vi "folder&single VI desc&help.vi"() -> ()   [LabVIEW 2020]
panel:
  in  "All / Selected by Name":bool
  in  "Same Desc":bool
  in  "Copy Descs to Tags":bool
  in  "PREV":bool
  in  "NEXT":bool
  out "filenames":string[](array[string])
  in  "Read entire Folder":bool
  in  "path":path
  in  "stop":bool
  in  "SAVE":bool
  in  "Copy Desc&Tags":bool
  in  "Same File":bool
  out "found index":i32[](array[numeric])
  in  "Select Name":string[](array[string])
  in  "Copy VI Descr W":bool
  in  "Tip W":string[](array[string])
  in  "Desc W":string[](array[string])
  out "Is Ind?":bool[](array[boolean])
  out "Desc":string[](array[string])
  out "Tip":string[](array[string])
  out "Name":string[](array[string])
  out "index":i32[](array[numeric])
  out "ClassID":u32[](array[numeric])
  out "ClassName":string[](array[string])
  in  "Generate Help Tag W":bool
  in  "Copy Help Tag":bool
  in  "Copy CHM path":bool
  in  "W vi path":path
  in  "Help:Document Path W":path
  in  "Help:Document Tag W":string
  in  "VI Description W":string
  out "VI Name W":string
  in  "Write":bool
  in  "Read":bool
  out "VI Name":string
  out "VI Description":string
  out "Help:Document Tag":string
  out "Help:Document Path":path
  in  "R vi path":path
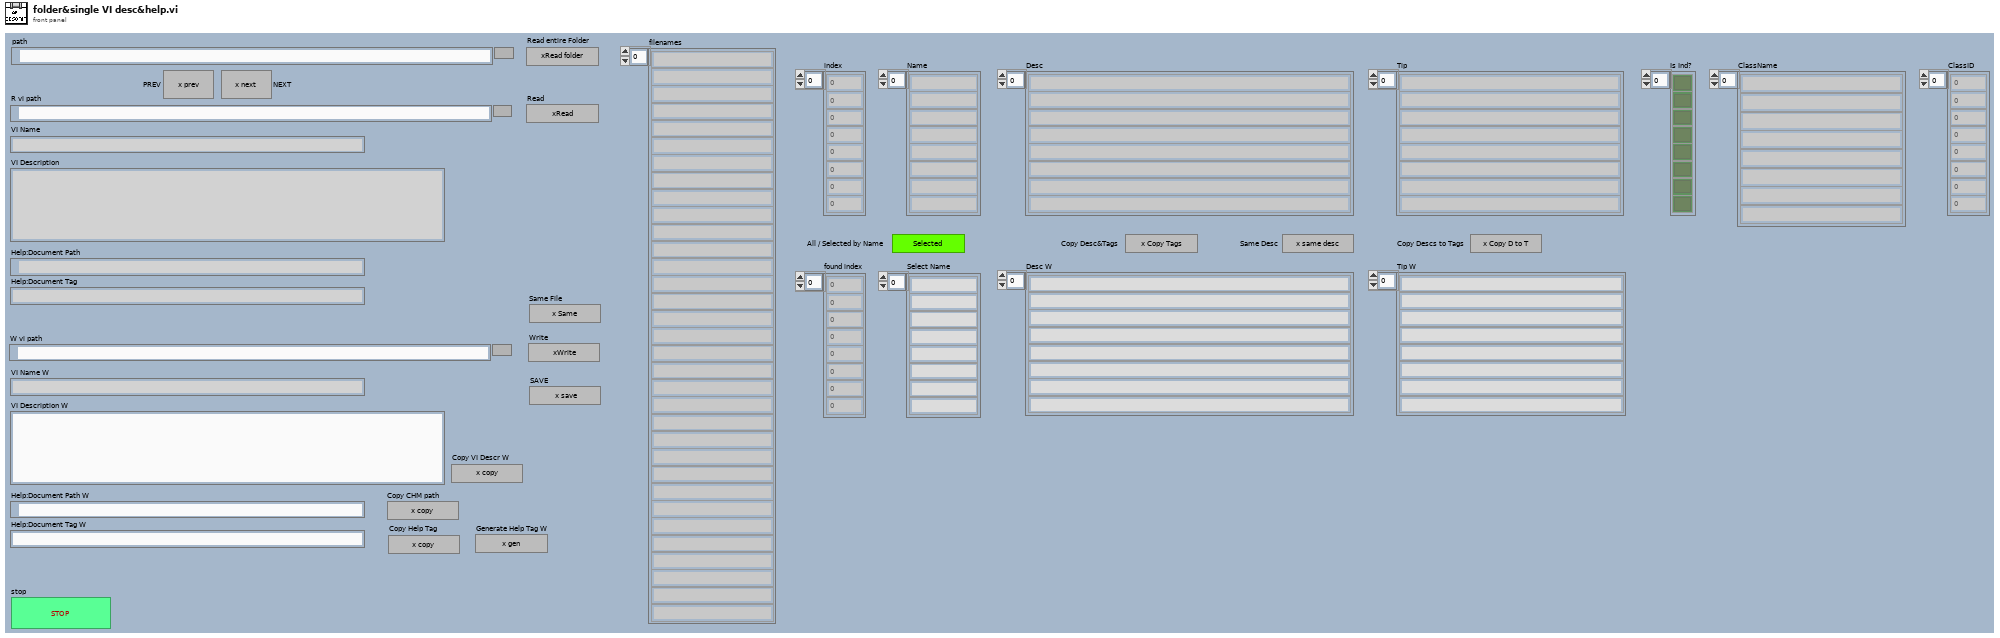
[diagram p1: front panel]
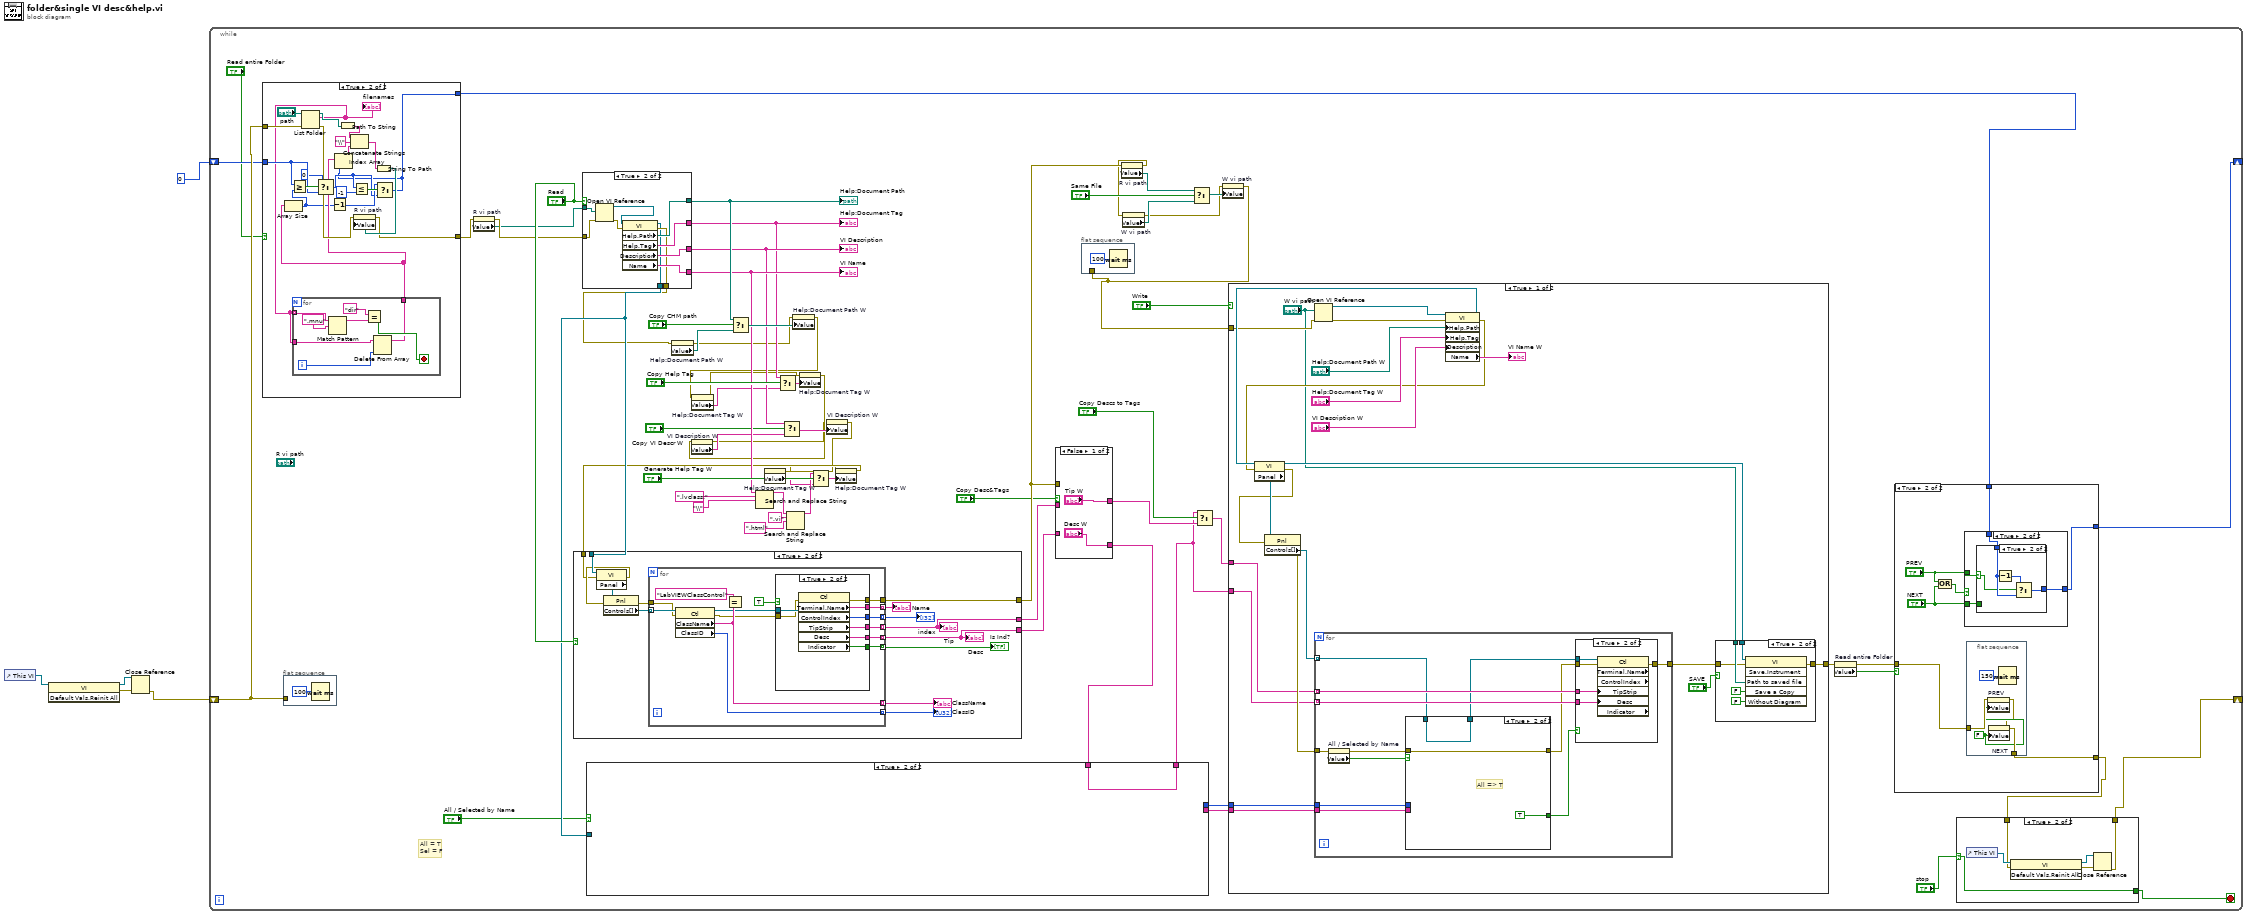
[diagram p0: block diagram]
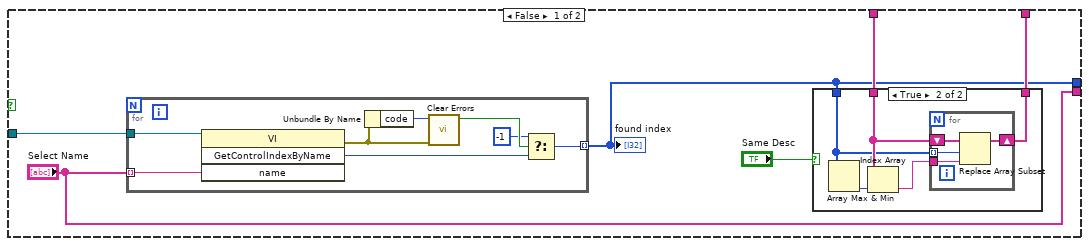
[diagram p2: hidden frame]
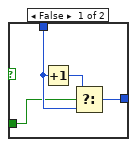
[diagram p8: hidden frame]
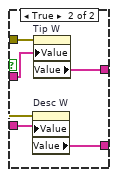
[diagram p9: hidden frame]
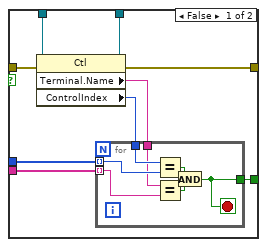
[diagram p11: hidden frame]
diagram:
  n1 = control-ref of="This VI"() -> (w4:refnum<vi>)
  n2 = invoke class="VI" method="Default Vals.Reinit All"(reference=w4) -> (reference out=w2:refnum<vi>, error out=w3:errorcluster)  [unwired: 2 in, 1 out]
  n3 = Close Reference(reference=w2, error in (no error)=w3) -> (error out=w1:errorcluster)
  n4 = while {
    shift-right: [w28] -> _
    shift-left: w1 -> [w72]
    shift-right: [w73] -> _
    shift-left: 0 -> [w71]
    stop <- w30 stop-if-true
    # "All = T\nSel = F"
    n5 = case shown="True" "Read entire Folder" {
      tunnel: w72 -> [w107 w122]
      tunnel: w71 -> [w108 w120]
      tunnel: [w108 w110] -> w70
      tunnel: [w107 w109] -> w37
      frame False {
      }
      frame True {
        n6 = List Folder(path="path", error in=w122) -> (path out=w128:path, filenames=w118:string[], error out=w125:errorcluster)  [unwired: 2 in, 1 out]
        "filenames" <- w118
        n7 = for {
          tunnel: w118 -> [w137] mode=indexing
          tunnel: w118 -> [w134]
          tunnel: [w130] -> w116
          i -> [w135]
          stop <- w131 stop-if-true
          n8 = Match Pattern(string=w137, regular expression=".mnu" ("string")) -> (before substring=w132:string)  [unwired: 1 in, 3 out]
          n9 = Equal?(x="dir" ("string"), y=w132) -> (x = y?=w131:bool)
          n10 = Delete From Array(array=w134, index=w135) -> (array with subset deleted=w130:string[])  [unwired: 1 in, 1 out]
        }
        n11 = Array Size(array=w116) -> (size(s)=w113:i32)
        n12 = Greater Or Equal?(x=w120, y=w113) -> (x >= y?=w121:bool)
        n13 = Select(t=0, s=w121, f=w120) -> (s? t:f=w111:i32)
        n14 = Decrement(x=w113) -> (x-1=w112:i32)
        n15 = Path To String(path=w128) -> (string=w127:string)
        n16 = Less Or Equal?(x=w111, y=-1) -> (x <= y?=w114:bool)
        n17 = Select(t=w112, s=w114, f=w111) -> (s? t:f=w110:i32)
        n18 = Index Array(array=w116, index=w110) -> (element=w117:string)
        n19 = Concatenate Strings(w127, "\\" ("string"), w117) -> (w126:string)
        n20 = String To Path(string=w126) -> (path=w124:path)
        n21 = property on="R vi path" class="Path"(error in=w125, "Value"=w124) -> (error out=w109:errorcluster)  [unwired: 1 in, 1 out]
      }
    }
    n22 = flat-sequence {
      tunnel: w72 -> [_]
      frame #0 {
        n23 = Wait (ms)(milliseconds to wait=u32 100) -> ()  [unwired: 1 out]
      }
    }
    n24 = property on="R vi path" class="Path"(error in=w37) -> (error out=w35:errorcluster, "Value"=w34:path)  [unwired: 1 in, 1 out]
    n25 = case shown="True" "Read" {
      tunnel: [_ w287] -> w65
      tunnel: [_ w286] -> w32
      tunnel: [_ w285] -> w50
      tunnel: [_ w284] -> w52
      tunnel: w35 -> [w277 w280]
      tunnel: [w277 w283] -> w19
      tunnel: w34 -> [_ w281]
      tunnel: [_ w278] -> w33
      frame False {
      }
      frame True {
        n26 = Open VI Reference(vi path=w281, error in (no error)=w280) -> (vi reference=w282:refnum<vi>, error out=w279:errorcluster)  [unwired: 4 in]
        n27 = property class="VI"(reference=w282, error in=w279) -> (reference out=w278:refnum<vi>, error out=w283:errorcluster, "Help.Path"=w287:path, "Help.Tag"=w286:string, "Description"=w285:string, "Name"=w284:string)
      }
    }
    "Help:Document Path" <- w65
    "Help:Document Tag" <- w32
    "VI Description" <- w50
    "VI Name" <- w52
    n28 = property on="Help:Document Path W" class="Path"(error in=w19) -> (error out=w18:errorcluster, "Value"=w63:path)  [unwired: 1 in, 1 out]
    n29 = Select(t=w65, s="Copy CHM path", f=w63) -> (s? t:f=w64:path)
    n30 = Search and Replace String(input string=w52, search string=".lvclass:", replace string="\\" ("replace string (\"\")")) -> (result string=w56:string)  [unwired: 5 in, 3 out]
    n31 = Search and Replace String(input string=w56, search string=".vi", replace string=".html" ("search string")) -> (result string=w53:string)  [unwired: 5 in, 3 out]
    n32 = property on="Help:Document Path W" class="Path"(error in=w18, "Value"=w64) -> (error out=w17:errorcluster)  [unwired: 1 in, 1 out]
    n33 = property on="Help:Document Tag W" class="Str"(error in=w17) -> (error out=w16:errorcluster, "Value"=w20:string)  [unwired: 1 in, 1 out]
    n34 = Select(t=w32, s="Copy Help Tag", f=w20) -> (s? t:f=w62:string)
    n35 = property on="Help:Document Tag W" class="Str"(error in=w16, "Value"=w62) -> (error out=w15:errorcluster)  [unwired: 1 in, 1 out]
    n36 = property on="VI Description W" class="Str"(error in=w15) -> (error out=w14:errorcluster, "Value"=w49:string)  [unwired: 1 in, 1 out]
    n37 = Select(t=w50, s="Copy VI Descr W", f=w49) -> (s? t:f=w48:string)
    n38 = property on="VI Description W" class="Str"(error in=w14, "Value"=w48) -> (error out=w12:errorcluster)  [unwired: 1 in, 1 out]
    n39 = property on="Help:Document Tag W" class="Str"(error in=w12) -> (error out=w11:errorcluster, "Value"=w10:string)  [unwired: 1 in, 1 out]
    n40 = Select(t=w53, s="Generate Help Tag W", f=w10) -> (s? t:f=w57:string)
    n41 = property on="Help:Document Tag W" class="Str"(error in=w11, "Value"=w57) -> (error out=w13:errorcluster)  [unwired: 1 in, 1 out]
    n42 = case shown="True" "Read" {
      tunnel: w33 -> [_ w254]
      tunnel: [w240 w244] -> w69
      tunnel: [_ w243] -> w68
      tunnel: [_ w242] -> w27
      tunnel: w13 -> [w240 w241]
      frame False {
      }
      frame True {
        n43 = property class="VI"(reference=w254, error in=w241) -> (error out=w245:errorcluster, "Panel"=w253:refnum<vi>)  [unwired: 1 out]
        n44 = property class="Pnl"(reference=w253, error in=w245) -> (error out=w246:errorcluster, "Controls[]"=w252:refnum<vi>[])  [unwired: 1 out]
        n45 = for {
          tunnel: w252 -> [w268] mode=indexing
          tunnel: [w265] -> w251 mode=indexing
          tunnel: [w267] -> w250 mode=indexing
          tunnel: [w263] -> w249 mode=indexing
          tunnel: [w262] -> w248 mode=indexing
          tunnel: [w261] -> w242 mode=indexing
          tunnel: [w260] -> w243 mode=indexing
          tunnel: [w258] -> w247 mode=indexing
          tunnel: w246 -> [w257]
          tunnel: [w255] -> w244
          n46 = property class="Ctl"(reference=w268, error in=w257) -> (reference out=w264:refnum<vi>, error out=w256:errorcluster, "ClassName"=w265:string, "ClassID"=w267:u32)
          n47 = Equal?(x="LabVIEWClassControl" ("search string"), y=w265) -> ()  [unwired: 1 out]
          n48 = case shown="True" TRUE {
            tunnel: w264 -> [_ w276]
            tunnel: [_ w271] -> w263
            tunnel: [_ w275] -> w262
            tunnel: [_ w274] -> w261
            tunnel: [_ w273] -> w260
            tunnel: [_ w272] -> w258
            tunnel: w256 -> [_ w270]
            tunnel: [_ w269] -> w255
            frame False {
            }
            frame True {
              n49 = property class="Ctl"(reference=w276, error in=w270) -> (error out=w269:errorcluster, "Terminal.Name"=w275:string, "ControlIndex"=w271:i32, "TipStrip"=w274:string, "Desc"=w273:string, "Indicator"=w272:bool)  [unwired: 1 out]
            }
          }
        }
        "ClassName" <- w251
        "ClassID" <- w250
        "index" <- w249
        "Name" <- w248
        "Tip" <- w242
        "Desc" <- w243
        "Is Ind?" <- w247
      }
    }
    n50 = case shown="False" "Copy Desc&Tags" {
      tunnel: w27 -> [_ w171]
      tunnel: w68 -> [_ w170]
      tunnel: w69 -> [_ w169]
      tunnel: ["Desc W" w168] -> w22
      tunnel: ["Tip W" w167] -> w25
      frame False {
      }
      frame True {
        n51 = property on="Desc W" class="Arr (strict)"(error in=w169, "Value"=w170) -> ("Value"=w168:string[])  [unwired: 1 in, 2 out]
        n52 = property on="Tip W" class="Arr (strict)"(error in=w169, "Value"=w171) -> ("Value"=w167:string[])  [unwired: 1 in, 2 out]
      }
    }
    n53 = case shown="True" "All / Selected by Name" {
      tunnel: w33 -> [w79 _]
      tunnel: ["Select Name" _] -> w23
      tunnel: w22 -> [w77 w98]
      tunnel: [w75 w98] -> w21
      tunnel: [w74 _] -> w7
      frame False {
        n54 = for {
          tunnel: w79 -> [w97]
          tunnel: "Select Name" -> [w91] mode=indexing
          tunnel: [w90] -> w74 mode=indexing
          n55 = invoke class="VI" method="GetControlIndexByName"(reference=w97, "name"=w91) -> (error out=w96:errorcluster, "GetControlIndexByName"=w93:i32)  [unwired: 2 in, 2 out]
          n56 = Unbundle By Name(w96) -> ("code"=w95:i32)
          n57 = call <vilib>:"Clear Errors.vi"("error in (no error)"=w96, "specific error code to clear (0: all)"=w95) -> ("specific error cleared?"=w94:bool)  [unwired: 4 in, 1 out]
          n58 = Select(t=-1, s=w94, f=w93) -> (s? t:f=w90:i32)
        }
        "found index" <- w74
        n59 = case shown="True" "Same Desc" {
          tunnel: w77 -> [w80 w85]
          tunnel: w74 -> [_ w83]
          tunnel: [w80 w82] -> w75
          frame False {
          }
          frame True {
            n60 = Array Max & Min(array=w83) -> (min index (indices)=w81:i32)  [unwired: 3 out]
            n61 = Index Array(array=w85, index=w81) -> (element=w84:string)
            n62 = for {
              tunnel: w84 -> [w88]
              tunnel: w83 -> [w87] mode=indexing
              shift-right: [w86] -> w82
              shift-left: w85 -> [w89]
              n63 = Replace Array Subset(array=w89, new element=w88, index=w87) -> (w86:string[])
            }
          }
        }
      }
      frame True {
      }
    }
    n64 = flat-sequence {
      tunnel: w39 -> [_]
      frame #0 {
        n65 = Wait (ms)(milliseconds to wait=u32 100) -> ()  [unwired: 1 out]
      }
    }
    n66 = property on="R vi path" class="Path"(error in=w69) -> (error out=w38:errorcluster, "Value"=w44:path)  [unwired: 1 in, 1 out]
    n67 = property on="W vi path" class="Path"(error in=w38) -> (error out=w41:errorcluster, "Value"=w43:path)  [unwired: 1 in, 1 out]
    n68 = Select(t=w44, s="Same File", f=w43) -> (s? t:f=w42:path)
    n69 = Select(t=w21, s="Copy Descs to Tags", f=w25) -> (s? t:f=w24:string[])
    n70 = property on="W vi path" class="Path"(error in=w41, "Value"=w42) -> (error out=w39:errorcluster)  [unwired: 1 in, 1 out]
    n71 = case shown="True" "Write" {
      tunnel: w39 -> [w179 w239]
      tunnel: [w173 w239] -> w9
      tunnel: w21 -> [w186 _]
      tunnel: w24 -> [w185 _]
      tunnel: w7 -> [w184 _]
      tunnel: w23 -> [w183 _]
      frame True {
        n72 = Open VI Reference(vi path="W vi path", error in (no error)=w179) -> (vi reference=w182:refnum<vi>, error out=w180:errorcluster)  [unwired: 4 in]
        n73 = property class="VI"(reference=w182, error in=w180, "Help.Path"="Help:Document Path W", "Help.Tag"="Help:Document Tag W", "Description"="VI Description W") -> (reference out=w181:refnum<vi>, error out=w178:errorcluster, "Name"=→"VI Name W":string)
        n74 = property class="VI"(reference=w181, error in=w178) -> (reference out=w176:refnum<vi>, error out=w187:errorcluster, "Panel"=w190:refnum<vi>)
        n75 = property class="Pnl"(reference=w190, error in=w187) -> (error out=w188:errorcluster, "Controls[]"=w189:refnum<vi>[])  [unwired: 1 out]
        n76 = for {
          tunnel: w189 -> [w205] mode=indexing
          tunnel: w185 -> [w213] mode=indexing
          tunnel: w186 -> [w212] mode=indexing
          tunnel: w188 -> [w204]
          tunnel: [w211] -> w174
          tunnel: w184 -> [w210]
          tunnel: w183 -> [w209]
          n77 = property on="All / Selected by Name" class="Bool (strict)"(error in=w204) -> (error out=w203:errorcluster, "Value"=w202:bool)  [unwired: 1 in, 1 out]
          n78 = case shown="True" w202 {
            tunnel: w210 -> [w222 _]
            tunnel: w209 -> [w221 _]
            tunnel: [w218 TRUE] -> w208
            tunnel: [w217 w231] -> w207
            tunnel: [w216 w232] -> w206
            tunnel: w205 -> [w215 w232]
            tunnel: w203 -> [w214 w231]
            frame False {
              n79 = property class="Ctl"(reference=w215, error in=w214) -> (reference out=w216:refnum<vi>, error out=w217:errorcluster, "Terminal.Name"=w220:string, "ControlIndex"=w219:i32)
              n80 = for {
                tunnel: w222 -> [w228] mode=indexing
                tunnel: w221 -> [w226] mode=indexing
                tunnel: w220 -> [w227]
                tunnel: w219 -> [w229]
                tunnel: [w223] -> w218
                stop <- w223 stop-if-true
                n81 = Equal?(x=w229, y=w228) -> (x = y?=w225:bool)
                n82 = Equal?(x=w227, y=w226) -> (x = y?=w224:bool)
                n83 = And(x=w225, y=w224) -> (x .and. y?=w223:bool)
              }
            }
            frame True {
              # "All => T"
            }
          }
          n84 = case shown="True" w208 {
            tunnel: w206 -> [_ w238]
            tunnel: w213 -> [_ w237]
            tunnel: w212 -> [_ w236]
            tunnel: w207 -> [w233 w235]
            tunnel: [w233 w234] -> w211
            frame False {
            }
            frame True {
              n85 = property class="Ctl" props=["Terminal", "Name", "ControlIndex", "TipStrip", "Desc", "Indicator"](reference=w238, error in=w235, "TipStrip"=w237, "Desc"=w236) -> (error out=w234:errorcluster)  [unwired: 4 out]
            }
          }
        }
        n86 = case shown="True" "SAVE" {
          tunnel: "W vi path" -> [_ w201]
          tunnel: w176 -> [_ w198]
          tunnel: w174 -> [w195 w197]
          tunnel: [w195 w196] -> w173
          frame False {
          }
          frame True {
            n87 = invoke class="VI" method="Save.Instrument"(reference=w198, error in=w197, "Path to saved file"=w201, "Save a Copy"=FALSE, "Without Diagram"=FALSE) -> (error out=w196:errorcluster)  [unwired: 1 in, 5 out]
          }
        }
      }
      frame False {
      }
    }
    n88 = property on="Read entire Folder" class="Bool (strict)"(error in=w9) -> (error out=w8:errorcluster, "Value"=w40:bool)  [unwired: 1 in, 1 out]
    n89 = case shown="True" w40 {
      tunnel: [w138 w146] -> w29
      tunnel: [w139 w145] -> w73
      tunnel: w70 -> [w139 w144]
      tunnel: w8 -> [w138 w140]
      frame False {
      }
      frame True {
        n90 = Or(x="PREV", y="NEXT") -> (x .or. y?=w142:bool)
        n91 = case shown="True" w142 {
          tunnel: [w147 w151] -> w145
          tunnel: w144 -> [w147 w150]
          tunnel: "PREV" -> [_ w149]
          tunnel: "NEXT" -> [_ w148]
          frame False {
          }
          frame True {
            n92 = case shown="True" w149 {
              selector: w149 -> [_ w156]
              tunnel: [w155 w159] -> w151
              tunnel: w150 -> [w154 w158]
              tunnel: w148 -> [w152 _]
              frame False {
                n93 = Increment(x=w154) -> (x+1=w153:i32)
                n94 = Select(t=w153, s=w152, f=w154) -> (s? t:f=w155:i32)
              }
              frame True {
                n95 = Decrement(x=w158) -> (x-1=w157:i32)
                n96 = Select(t=w157, s=w156, f=w158) -> (s? t:f=w159:i32)
              }
            }
          }
        }
        n97 = flat-sequence {
          tunnel: w140 -> [w162]
          tunnel: [w164] -> w146
          frame #0 {
            w161 = FALSE ("NEXT")
            n98 = property on="PREV" class="Bool (strict)"(error in=w162, "Value"=w161) -> (error out=w160:errorcluster)  [unwired: 1 in, 1 out]
            n99 = property on="NEXT" class="Bool (strict)"(error in=w160, "Value"=w161) -> (error out=w164:errorcluster)  [unwired: 1 in, 1 out]
            n100 = Wait (ms)(milliseconds to wait=u32 150) -> ()  [unwired: 1 out]
          }
        }
      }
    }
    n101 = case shown="True" "stop" {
      selector: "stop" -> [w100 w103]
      tunnel: [w100 w103] -> w30
      tunnel: w29 -> [w99 w102]
      tunnel: [w99 w101] -> w28
      frame False {
      }
      frame True {
        n102 = control-ref of="This VI"() -> (w106:refnum<vi>)
        n103 = invoke class="VI" method="Default Vals.Reinit All"(reference=w106, error in=w102) -> (reference out=w104:refnum<vi>, error out=w105:errorcluster)  [unwired: 1 in, 1 out]
        n104 = Close Reference(reference=w104, error in (no error)=w105) -> (error out=w101:errorcluster)
      }
    }
  }
